vi "Q8381 QRY GRAPH DATA POINT OUT.vi"(2 "GPIB address":u16=8 max=31 step=1, 3 "VISA resource name":refnum<visa-resource-name>) -> (0 "Data point":u16, 1 "GPIB status":bool)   [LabVIEW 2017]
panel:
  out "Program code":string
  # "Read graph data point"
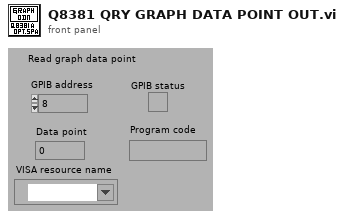
[diagram p1: front panel]
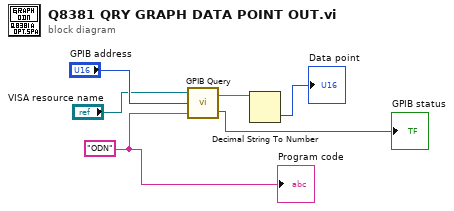
[diagram p0: block diagram]
diagram:
  w3 = "ODN"
  n1 = call "GPIB Query.vi"("Command String"=w3, "Address"="GPIB address", "VISA resource name"="VISA resource name") -> ("Error"=→"GPIB status":bool, "Query Data"=w5:string)
  n2 = Decimal String To Number(string=w5) -> (number=→"Data point":i32)  [unwired: 2 in, 1 out]
  "Program code" <- w3
